vi "CC Observation Calculate Circular Dither Points.vi"(8 "error in (no error)":errorcluster, 11 "Dither Options":T2) -> (0 "error out":errorcluster, 3 "Points":T1[](array[typedef]))   [LabVIEW 2024]
uses:
  typedefs/CC cluster Observation Dither Options.ctl
  typedefs/CC enum Dither Selection.ctl
  typedefs/CC Dithering Offsets.ctl
panel:
  out "XY Graph":cluster{"X":dbl, "Y":dbl}[](graph)
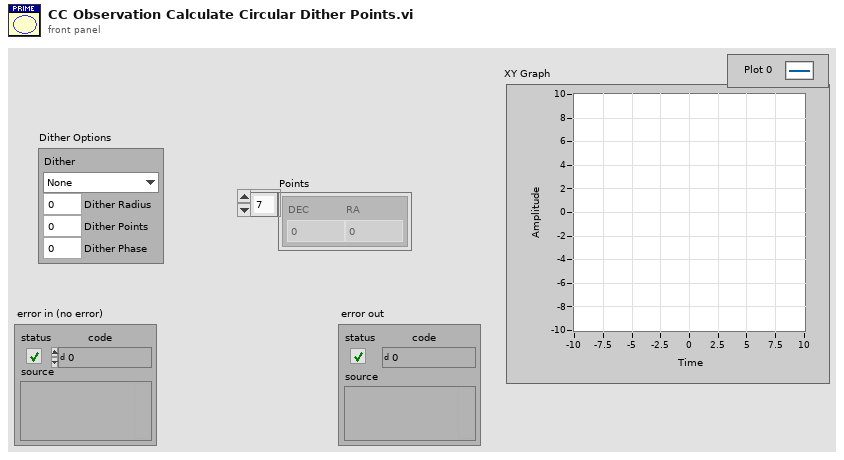
[diagram p1: front panel]
types:
  T1 = typedef "CC Dithering Offsets.ctl" = cluster{"DEC":dbl, "RA":dbl}
  T2 = typedef "CC cluster Observation Dither Options.ctl" = cluster{"Dither":T3, "Dither Radius":dbl, "Dither Points":i32, "Dither Phase":dbl}
  T3 = typedef "CC enum Dither Selection.ctl" = enum16{"None", "Circle", "Random"}
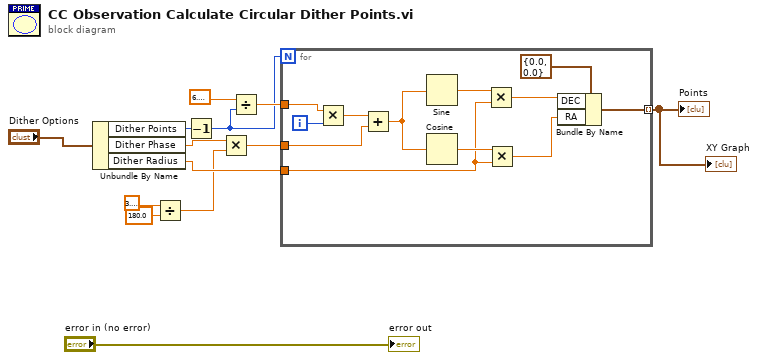
[diagram p0: block diagram]
diagram:
  n1 = Unbundle By Name("Dither Options") -> ("Dither Points"=w9:i32, "Dither Phase"=w8:dbl, "Dither Radius"=w7:dbl)
  n2 = Divide(x=3.141592653589793, y=180.0) -> (x/y=w2:dbl)
  n3 = Decrement(x=w9) -> (x-1=w1:i32)
  n4 = Multiply(x=w8, y=w2) -> (x*y=w5:dbl)
  n5 = Divide(x=6.283185307179586, y=w1) -> (x/y=w11:dbl)
  n6 = for {
    N: w1 -> [_]
    tunnel: w11 -> [w24]
    tunnel: w5 -> [w22]
    tunnel: w7 -> [w18]
    tunnel: [w14] -> w6 mode=indexing
    i -> [w25]
    n7 = Multiply(x=w24, y=w25) -> (x*y=w23:dbl)
    n8 = Add(x=w23, y=w22) -> (x+y=w21:dbl)
    n9 = Sine(x=w21) -> (sin(x)=w19:dbl)
    n10 = Cosine(x=w21) -> (cos(x)=w20:dbl)
    n11 = Multiply(x=w19, y=w18) -> (x*y=w16:dbl)
    n12 = Multiply(x=w20, y=w18) -> (x*y=w15:dbl)
    n13 = Bundle By Name(cluster=T1 {"DEC"=0.0, "RA"=0.0} ("element"), "DEC"=w16, "RA"=w15) -> (w14:T1)
  }
  "XY Graph" <- w6
  "Points" <- w6
  "error out" <- "error in (no error)"
